vi "communicateMLCRun.vi"(8 "error in (no error)":errorcluster) -> (0 "error out":errorcluster)   [LabVIEW 2017, in "communicateMLC.lvlib"]
doc: "This VI contains the loop which controls external communication to the PC, which is achieved by UDP. The module loop does not start unitl the 'start' command is received from the Program Control Module."
uses:
  communicateMLC.lvlib
  UEFGV/Type Def/UEFGV_States.ctl
  TypeDefs/LoopStates.ctl
  ErrorMonitor/ErrorMonitor.lvlib
  loggingModule/loggingModule.lvlib
panel:
  out "shutdown":bool
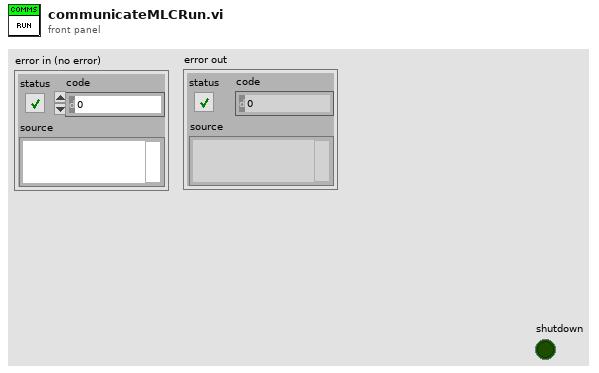
[diagram p1: front panel]
types:
  T1 = typedef "UEFGV_States.ctl" = enum16{"Create", "Get", "Destroy"}
  T2 = typedef "LoopStates.ctl" = enum16{"start", "wait", "run", "end"}
  T3 = typedef "dataOut.ctl" = cluster{"X0pos":dbl, "Y0pos":dbl, "Z0pos":dbl, "Fx":dbl, "Fy":dbl, "Fz":dbl, "Encoder1":i32, "Encoder2":i32, "Pot1":dbl, "Pot2":dbl, "Theta0":dbl, "Theta1":dbl, "X1pos":dbl, "Y1pos":dbl, "Z1pos":dbl, "X2pos":dbl, "Y2pos":dbl, "Z2pos":dbl, "ErrorOccurred":bool}
  T4 = typedef "dataIn.ctl" = cluster{"Xtarget":dbl, "Ytarget":dbl, "Ztarget":dbl, "X_Attractor 1":dbl, "Y_Attractor 1":dbl, "Z_Attractor 1":dbl, "X_Attractor 2":dbl, "Y_Attractor 2":dbl, "Z_Attractor 2":dbl, "Traj Flag":bool, "DeadZone":dbl, "Assistance":bool, "Shutdown?":bool, "AssistanceLevel":dbl}
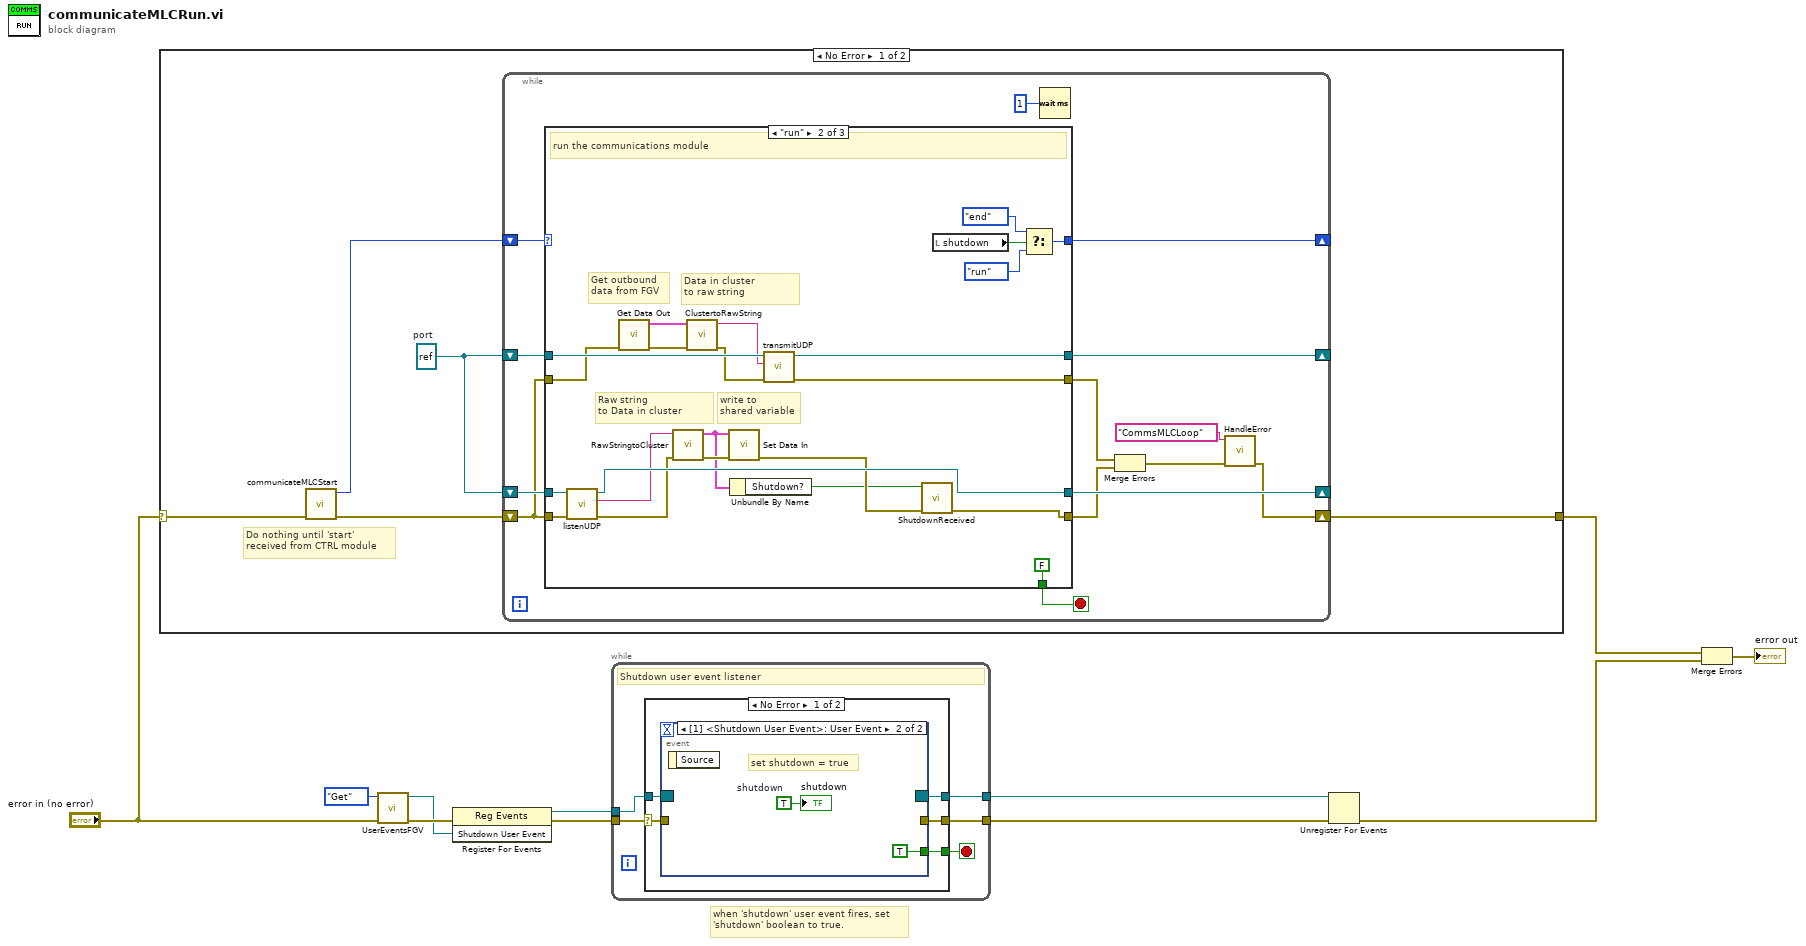
[diagram p0: block diagram]
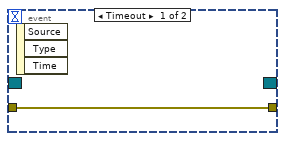
[diagram p2: hidden frame]
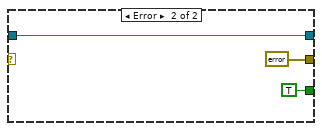
[diagram p3: hidden frame]
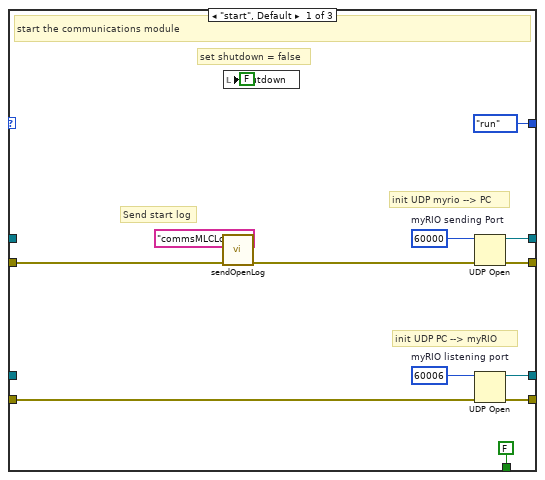
[diagram p4: hidden frame]
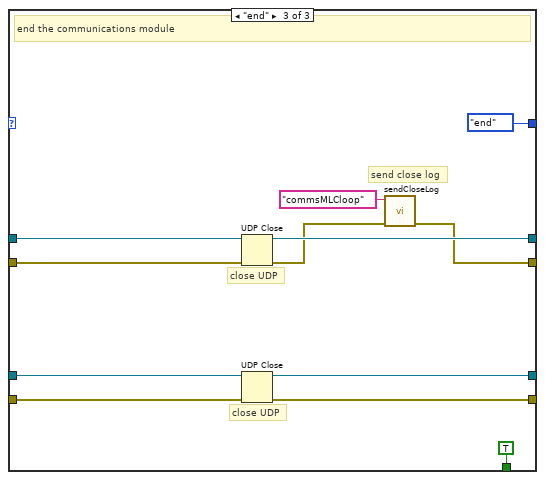
[diagram p5: hidden frame]
diagram:
  # "when 'shutdown' user event fires, set\n'shutdown' boolean to true."
  n1 = case shown="No Error" "error in (no error)" {
    selector: "error in (no error)" -> [w16 w79]
    tunnel: [w12 w79] -> w3
    frame No Error {
      w14 = refnum<k16> refnum  # port
      # "Do nothing until 'start'\nreceived from CTRL module"
      n2 = call "communicateMLCStart.vi"("error in (no error)"=w16) -> ("error out"=w13:errorcluster, "message out"=w15:T2)  [unwired: 9 in]
      n3 = while {
        shift-right: [w28] -> _
        shift-left: w15 -> [w30]
        shift-right: [w26] -> _
        shift-left: w14 -> [w23]
        shift-right: [w25] -> _
        shift-left: w14 -> [w24]
        shift-right: [w17] -> w12
        shift-left: w13 -> [w20]
        stop <- w29 stop-if-true
        n4 = case shown="\"run\"" w30 {
          tunnel: [FALSE FALSE TRUE] -> w29
          tunnel: [LoopStates."run" ("message out") w57 LoopStates."end" ("message out")] -> w28
          tunnel: [w40 w63 w74] -> w26
          tunnel: [w38 w61 w76] -> w25
          tunnel: w20 -> [w37 w64 w73]
          tunnel: [w36 w60 w69] -> w22
          tunnel: [w35 w46 w72] -> w21
          tunnel: w24 -> [_ w62 w77]
          tunnel: w23 -> [_ w65 w75]
          tunnel: w20 -> [w31 w49 w67]
          frame "start", Default {
            w39 = u16 60000  # myRIO sending Port
            w41 = u16 60006  # myRIO listening port
            # "Send start log"
            # "set shutdown = false"
            # "init UDP PC --> myRIO"
            # "init UDP myrio --> PC"
            # "start the communications module"
            n5 = call "sendOpenLog.vi"("error in (no error)"=w31, "source"="commsMLCLoop") -> ("error out"=w32:errorcluster)  [unwired: 9 in]
            n6 = local write "shutdown"(FALSE ("shutdown")) -> ()
            n7 = UDP Open(8:w32, 11:w39) -> (port=w38:refnum<k16>, 0:w36:errorcluster)  [unwired: 3 in, 1 out]
            n8 = UDP Open(8:w37, 11:w41) -> (port=w40:refnum<k16>, 0:w35:errorcluster)  [unwired: 3 in, 1 out]
          }
          frame "run" {
            # "Data in cluster\nto raw string"
            # "Raw string\nto Data in cluster"
            # "Get outbound \ndata from FGV"
            # "write to \nshared variable"
            # "run the communications module"
            n9 = call "listenUDP.vi"("error in (no error)"=w64, "UDP Network Connection in"=w65) -> ("error out"=w55:errorcluster, "data out"=w54:string, "UDP Network Connection out"=w63:refnum<k16>)  [unwired: 7 in]
            n10 = call "Get Data Out.vi"("error in (no error)"=w49) -> ("error out"=w52:errorcluster, "DataOut"=w53:T3)  [unwired: 9 in]
            n11 = call "RawStringtoCluster.vi"("error in (no error)"=w55, "Raw String"=w54) -> ("error out"=w56:errorcluster, "DataIn"=w48:T4)  [unwired: 8 in]
            n12 = call "ClustertoRawString.vi"("error in (no error)"=w52, "DataOut"=w53) -> ("error out"=w51:errorcluster, "DataOutstring"=w50:string)  [unwired: 8 in]
            n13 = call "Set Data In.vi"("error in (no error)"=w56, "DataIn"=w48) -> ("error out"=w47:errorcluster)  [unwired: 9 in]
            n14 = Unbundle By Name(w48) -> ("Shutdown?"=w45:bool)
            n15 = call "transmitUDP.vi"("error in (no error)"=w51, "data in"=w50, "UDP Network Connection in"=w62) -> ("error out"=w60:errorcluster, "UDP Network Connection out"=w61:refnum<k16>)  [unwired: 7 in]
            n16 = call "ShutdownReceived.vi"("error in (no error)"=w47, "Shutdown?"=w45) -> ("error out"=w46:errorcluster)  [unwired: 9 in]
            n17 = local read "shutdown"() -> (w59:bool)
            n18 = Select(t=LoopStates."end" ("message out"), s=w59, f=LoopStates."run" ("message out")) -> (s? t:f=w57:T2)
          }
          frame "end" {
            # "send close log"
            # "close UDP"
            # "close UDP"
            # "end the communications module"
            n19 = UDP Close(connection ID=w77, 8:w67) -> (connection ID out=w76:refnum<k16>, error out=w70:errorcluster)
            n20 = UDP Close(connection ID=w75, 8:w73) -> (connection ID out=w74:refnum<k16>, error out=w72:errorcluster)
            n21 = call "sendCloseLog.vi"("error in (no error)"=w70, "Source"="commsMLCloop") -> ("error out"=w69:errorcluster)  [unwired: 9 in]
          }
        }
        n22 = Wait (ms)(milliseconds to wait=u32 1) -> ()  [unwired: 1 out]
        n23 = Merge Errors(w22, w21) -> (w18:errorcluster)
        n24 = call "HandleError.vi"("error in (no error)"=w18, "Source"="CommsMLCLoop") -> ("error out"=w17:errorcluster)  [unwired: 9 in]
      }
    }
    frame Error {
    }
  }
  n25 = call "UserEventsFGV.vi"("error in (no error)"="error in (no error)", "Command"=UEFGV_States."Get") -> ("error out"=w9:errorcluster, "Shutdown User Event"=w8:refnum<user-event>)  [unwired: 8 in]
  n26 = register-events(error in=w9, w8) -> (reference out=w11:refnum<event-registration>, error out=w6:errorcluster)  [unwired: 1 in]
  n27 = while {
    tunnel: w11 -> [w84]
    tunnel: [w83] -> w10
    tunnel: w6 -> [w81]
    tunnel: [w80] -> w7
    stop <- w82 stop-if-true
    # "Shutdown user event listener"
    n28 = case shown="No Error" w81 {
      selector: w81 -> [w86 _]
      tunnel: w84 -> [w89 w94]
      tunnel: [w88 w94] -> w83
      tunnel: [w87 TRUE] -> w82
      tunnel: [w85 errorcluster {"status"=FALSE, "code"=0, "source"=""} ("error out")] -> w80
      frame No Error {
        n29 = event shown="[1] <Shutdown User Event>: User Event" {
          selector: w89 -> [_ _]
          dyn-events: [_ _] -> w88
          timeout: _ -> [_ _]
          tunnel: w86 -> [w90 _]
          tunnel: [w90 _] -> w85
          tunnel: [_ TRUE] -> w87
          event Timeout {
            n30 = event-data() -> ()  [unwired: 1 in, 3 out]
          }
          event User Event {
            w91 = TRUE  # shutdown
            # "set shutdown = true"
            n31 = event-data() -> ()  [unwired: 1 in, 1 out]
            "shutdown" <- w91
          }
        }
      }
      frame Error {
      }
    }
  }
  n32 = Unregister For Events(event registration refnum=w10, error in=w7) -> (error out=w4:errorcluster)
  n33 = Merge Errors(w3, w4) -> (→"error out":errorcluster)
